vi "auto_adjust.vi"(11 "NavData Out 2":T1) -> (3 "output cluster":cluster{"Change amount\n":dbl, dbl, i32, i32})   [LabVIEW 2015]
uses:
  <vilib>/LVH/AR Drone Toolkit/Decode NavData/Typedefs/NavData Demo.ctl
  <vilib>/LVH/AR Drone Toolkit/AR Drone.lvlib
panel:
  in  "Numeric 3":dbl
  in  "Change amount":dbl
  in  "Viteza Threshold":dbl
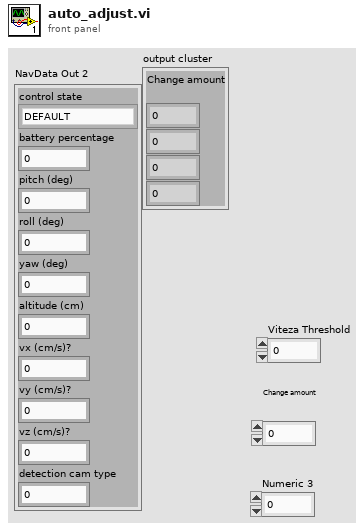
[diagram p1: front panel]
types:
  T1 = typedef "AR Drone.lvlib/NavData Demo.ctl" = cluster{"control state":enum32{"DEFAULT", "INIT", "LANDING", "FLYING", "HOVERING", "TEST", "TRANS_TAKEOFF", "TRANS_GOTOFIX", "TRANS_LANDING"}, "battery percentage":u32, "pitch (deg)":sgl, "roll (deg)":sgl, "yaw (deg)":sgl, "altitude (cm)":u32, "vx (cm/s)?":sgl, "vy (cm/s)?":sgl, "vz (cm/s)?":sgl, "detection cam type":u32}
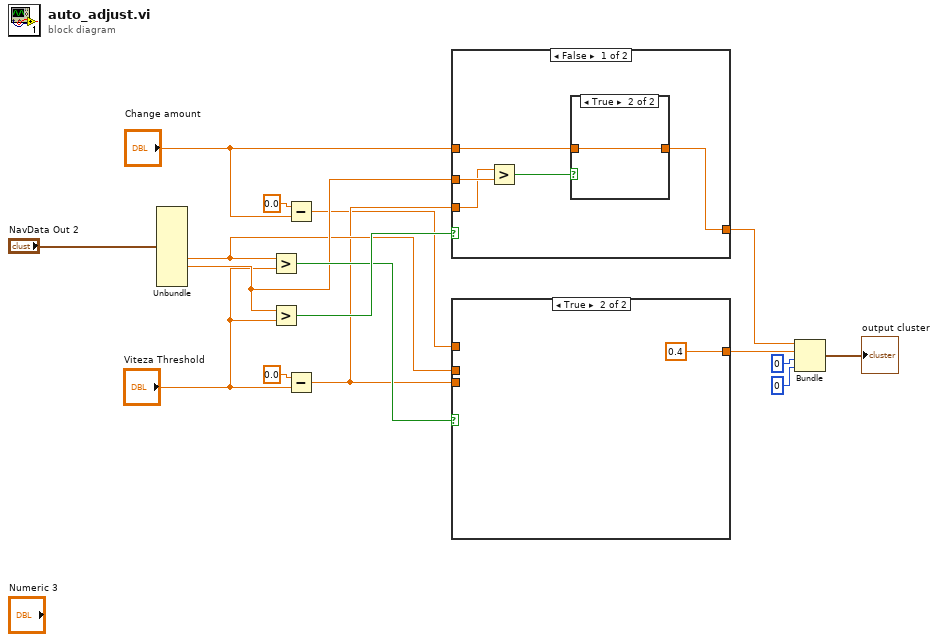
[diagram p0: block diagram]
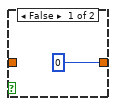
[diagram p2: hidden frame]
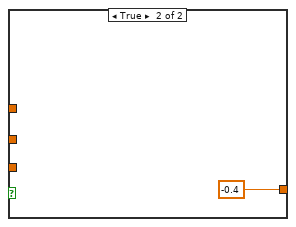
[diagram p3: hidden frame]
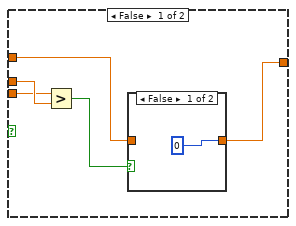
[diagram p4: hidden frame]
diagram:
  n1 = Unbundle("NavData Out 2") -> ("vx (cm/s)?"=w12:sgl, "vy (cm/s)?"=w13:sgl)  [unwired: 8 out]
  n2 = Greater?(x=w12, y="Viteza Threshold") -> (0:w14:bool)
  n3 = Greater?(x=w13, y="Viteza Threshold") -> (0:w15:bool)
  n4 = Subtract(x=0.0, y="Change amount") -> (x-y=w3:dbl)
  n5 = Subtract(x=0.0, y="Viteza Threshold") -> (x-y=w5:dbl)
  n6 = case shown="False" w15 {
    tunnel: [w20 -0.4] -> w11
    tunnel: w13 -> [w19 _]
    tunnel: w5 -> [w18 _]
    tunnel: "Change amount" -> [w17 _]
    frame False {
      n7 = Greater?(x=w18, y=w19) -> (0:w21:bool)
      n8 = case shown="True" w21 {
        tunnel: [0 w23] -> w20
        tunnel: w17 -> [_ w23]
        frame False {
        }
        frame True {
        }
      }
    }
    frame True {
    }
  }
  n9 = case shown="True" w14 {
    tunnel: [w27 0.4] -> w8
    tunnel: w12 -> [w28 _]
    tunnel: w5 -> [w26 _]
    tunnel: w3 -> [w25 _]
    frame False {
      n10 = Greater?(x=w26, y=w28) -> (0:w29:bool)
      n11 = case shown="False" w29 {
        tunnel: [0 w31] -> w27
        tunnel: w25 -> [_ w31]
        frame False {
        }
        frame True {
        }
      }
    }
    frame True {
    }
  }
  n12 = Bundle("Change amount"=w11, w8, 0, 0) -> (→"output cluster":cluster{"Change amount\n":dbl, dbl, i32, i32})  [unwired: 1 in]
